vi "ResetAutoshotButton.vi"(11 "Buttons":bool[](array[boolean])) -> ()   [LabVIEW 2015]
uses:
  Utilities/GeneralGlobals.vi
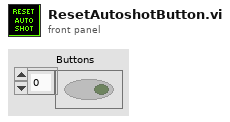
[diagram p1: front panel]
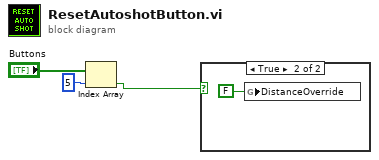
[diagram p0: block diagram]
diagram:
  n1 = Index Array(array="Buttons", index=5) -> (element=w1:bool)
  n2 = case shown="True" w1 {
    frame False {
    }
    frame True {
      n3 = global write "GeneralGlobals.vi" "DistanceOverride"(FALSE ("DistanceOverride")) -> ()
    }
  }
